vi "Configure Measurement Histogram (Setup And Hold).vi"(0 "VISA resource name":refnum<visa-resource-name>, 1 "Enable Measurement Histogram (Enable)":bool, 2 "Clock Source (2: Channel 2)":i32(ring) items=["Channel 1", "Channel 2", "Channel 3", "Channel 4", "Function 1", "Function 2", "Function 3", "Function 4", "Memory 1", "Memory 2", "Memory 3", "Memory 4"], 3 "Clock Source Direction (0: Rising)":i32(ring) items=["Rising", "Falling"], 5 "Data Source (1: Channel 1)":i32(ring) items=["Channel 1", "Channel 2", "Channel 3", "Channel 4", "Function 1", "Function 2", "Function 3", "Function 4", "Memory 1", "Memory 2", "Memory 3", "Memory 4"], 7 "Data Source Direction (0: Rising)":i32(ring) items=["Rising", "Falling", "Both"], 9 "Measurement Function (0: Setup Time)":i32(ring) items=["Setup Time", "Hold Time"], 11 "error in (no error)":errorcluster) -> (4 "VISA resource name out":refnum<visa-resource-name>, 15 "error out":errorcluster)   [LabVIEW 2009, in "Agilent 8000 Series.lvlib"]
doc: "Configures the Setup time/Hold time measurement and enables the Measurement Histogram Jitter analysis on it.\n\n<B>Note:</B>\nCalling this VI disables all previously enabled measurements and clears existing measurement results from display."
uses:
  Agilent 8000 Series.lvlib
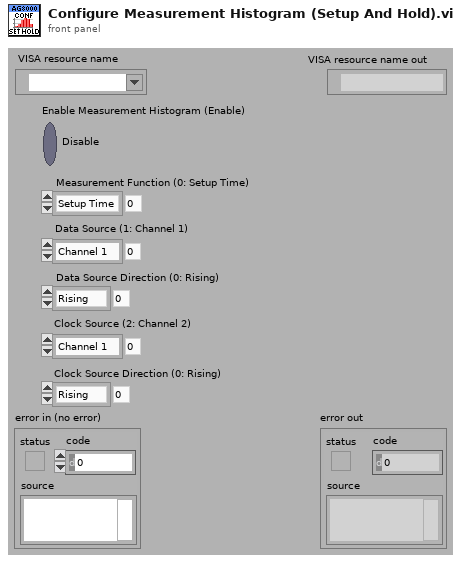
[diagram p1: front panel]
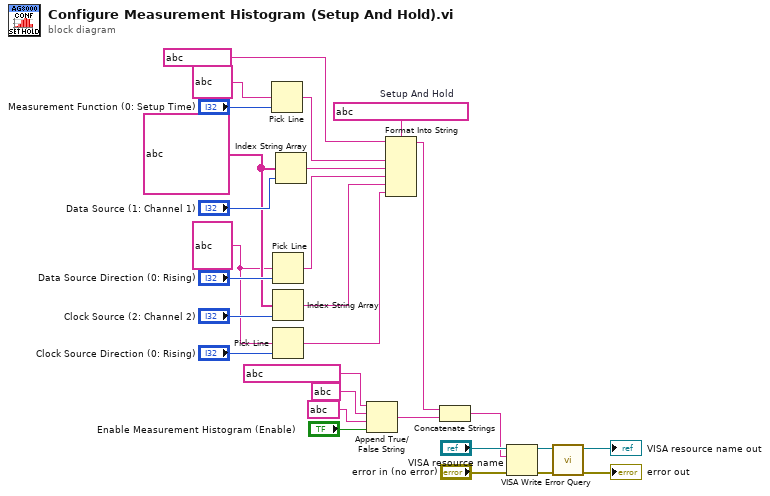
[diagram p0: block diagram]
diagram:
  w14 = string ?  # Setup And Hold
  w15 = string ? ("multi-line string")
  w18 = string[] ?
  n1 = Pick Line(multi-line string=string ?, line index="Measurement Function (0: Setup Time)") -> (output string=w13:string)  [unwired: 1 in]
  n2 = Pick Line(multi-line string=w15, line index="Data Source Direction (0: Rising)") -> (output string=w11:string)  [unwired: 1 in]
  n3 = Index String Array(1:"Clock Source (2: Channel 2)", 2:w18) -> (0:w10:string)  [unwired: 1 in]
  n4 = Pick Line(multi-line string=w15, line index="Clock Source Direction (0: Rising)") -> (output string=w9:string)  [unwired: 1 in]
  n5 = Index String Array(1:"Data Source (1: Channel 1)", 2:w18) -> (0:w12:string)  [unwired: 1 in]
  n6 = Append True/False String(1:"Enable Measurement Histogram (Enable)", 2:string ? ("false string"), 3:string ? ("true string"), 4:string ? ("string (\"\")")) -> (0:w2:string)
  n7 = Format Into String(format string=w14, initial string=string ?, w13, w12, w11, w10, w9) -> (resulting string=w3:string)  [unwired: 1 in, 1 out]
  n8 = Concatenate Strings(w3, w2) -> (w1:string)
  n9 = VISA Write(VISA resource name="VISA resource name", write buffer=w1, error in (no error)="error in (no error)") -> (VISA resource name out=w24:refnum<visa-resource-name>, error out=w23:errorcluster)  [unwired: 1 out]
  n10 = call "Error Query.vi"("error in (no error)"=w23, "VISA resource name"=w24) -> ("error out"=→"error out":errorcluster, "VISA resource name out"=→"VISA resource name out":refnum<visa-resource-name>)  [unwired: 6 in, 2 out]
